vi "Check Status.vi"(8 "error in (no error)":errorcluster, 11 "Fluke Multimeter in":refnum<class "Fluke Multimeter.lvclass">) -> (0 "error out":errorcluster, 1 "Status":string, 2 "Ready?":bool, 3 "Fluke Multimeter out":refnum<class "Fluke Multimeter.lvclass">)   [LabVIEW 2012, in "Fluke Multimeter.lvclass"]
doc: "(Dynamic) Check if the instrument is powered on and update its member data with the instrument's current status. Optionally return a text status message."
uses:
  Fluke Multimeter.lvclass
  Utility Classes/Readable/Readable.lvclass
  Fluke Multimeter.lvclass/Fluke Multimeter.ctl
  Fluke 8840/Fluke 8840.lvlib
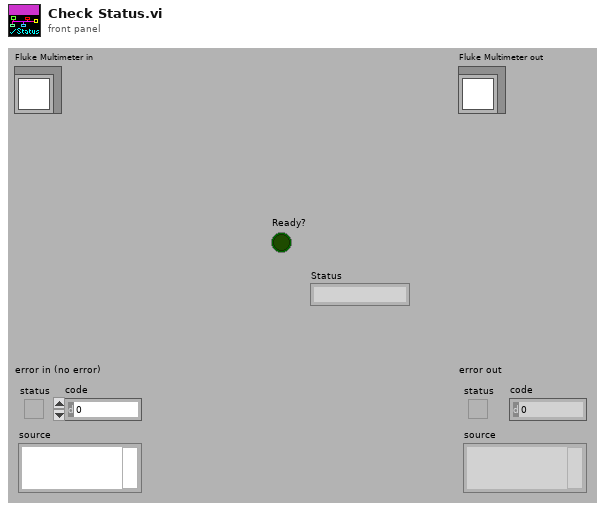
[diagram p1: front panel]
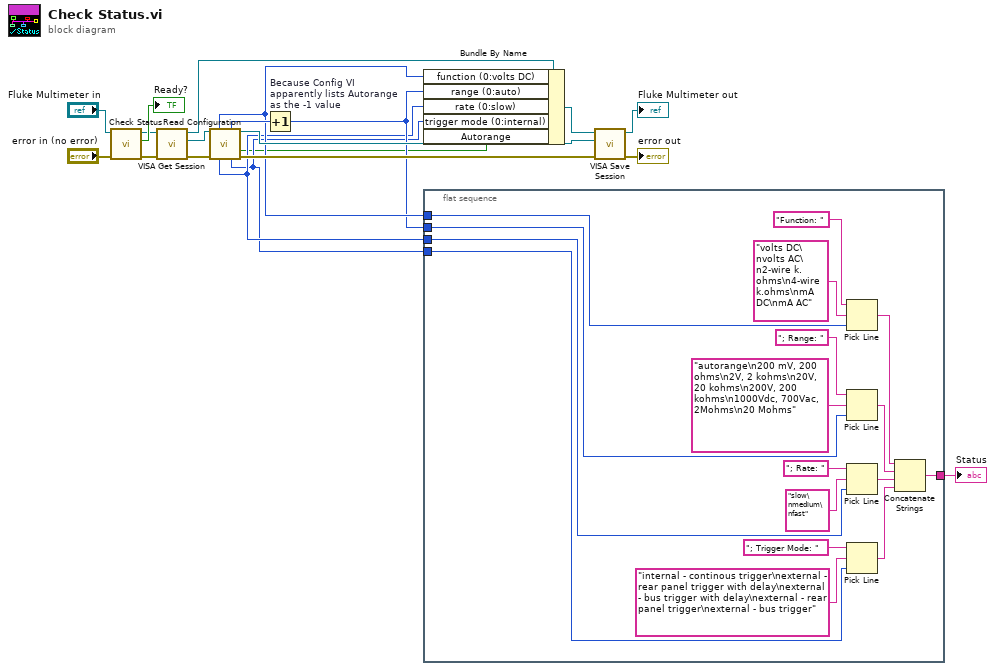
[diagram p0: block diagram]
diagram:
  n1 = call-parent "Check Status.vi"("error in (no error)"="error in (no error)", "Instrument in"="Fluke Multimeter in") -> ("error out"=w7:errorcluster, "Ready?"=→"Ready?":bool, "Instrument out"=w16:refnum<class "Fluke Multimeter.lvclass">)  [unwired: 7 out]
  n2 = call-dynamic "VISA Get Session.vi"("error in (no error)"=w7, "Instrument.lvclass in"=w16) -> ("error out"=w6:errorcluster, "VISA Resource Name"=w10:refnum<visa-resource-name>, "Instrument.lvclass out"=w13:refnum<class "Fluke Multimeter.lvclass">)  [unwired: 7 out]
  n3 = call "Read Configuration.vi"("VISA resource name"=w10, "error in (no error)"=w6) -> ("function"=w5:i32, "range"=w11:i32, "VISA resource name out"=w8:refnum<visa-resource-name>, "autorange"=w1:bool, "rate"=w3:i32, "trigger mode"=w2:i32, "error out"=w9:errorcluster)  [unwired: 7 out]
  n4 = Increment "Because Config VI\napparently lists Autorange\nas the -1 value"(x=w11) -> (x+1=w4:i32)
  n5 = Bundle By Name(cluster=w13, "function (0:volts DC)"=w5, "range (0:auto)"=w4, "rate (0:slow)"=w3, "trigger mode (0:internal)"=w2, "Autorange"=w1) -> (w12:refnum<class "Fluke Multimeter.lvclass">)
  n6 = flat-sequence {
    tunnel: [w35] -> w17
    tunnel: w5 -> [w33]
    tunnel: w4 -> [w30]
    tunnel: w3 -> [w25]
    tunnel: w2 -> [w24]
    frame #0 {
      n7 = Pick Line(string ("")="Function: ", multi-line string="volts DC\nvolts AC\n2-wire k.ohms\n4-wire k.ohms\nmA DC\nmA AC", line index=w33) -> (output string=w36:string)
      n8 = Pick Line(string ("")="; Range: ", multi-line string="autorange\n200 mV, 200 ohms\n2V, 2 kohms\n20V, 20 kohms\n200V, 200 kohms\n1000Vdc, 700Vac, 2Mohms\n20 Mohms", line index=w30) -> (output string=w29:string)
      n9 = Pick Line(string ("")="; Rate: ", multi-line string="slow\nmedium\nfast", line index=w25) -> (output string=w22:string)
      n10 = Pick Line(string ("")="; Trigger Mode: ", multi-line string="internal - continous trigger\nexternal - rear panel trigger with delay\nexternal - bus trigger with delay\nexternal - rear panel trigger\nexternal - bus trigger", line index=w24) -> (output string=w21:string)
      n11 = Concatenate Strings(w36, w29, w22, w21) -> (w35:string)
    }
  }
  n12 = call-dynamic "VISA Save Session.vi"("error in (no error)"=w9, "VISA Resource Name"=w8, "Instrument.lvclass in"=w12) -> ("error out"=→"error out":errorcluster, "Instrument.lvclass out"=→"Fluke Multimeter out":refnum<class "Fluke Multimeter.lvclass">)  [unwired: 7 out]
  "Status" <- w17
